vi "Generate data string.vi"(7 "New file":bool, 10 "Speed window data":T1, 11 "Timestamp at trial start":timestamp) -> (1 "Data String":string, 3 "Timestamp at trial start":timestamp)   [LabVIEW 2020]
uses:
  Typedefs/Speed window notifier data.ctl
  Typedefs/Speed logging states enum.ctl
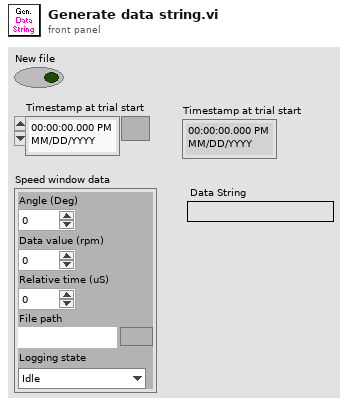
[diagram p1: front panel]
types:
  T1 = typedef "Speed window notifier data.ctl" = cluster{"Angle (Deg)":dbl, "Data value (rpm)":dbl, "Relative time (uS)":i32, "File path":path, "Logging state":T2}
  T2 = typedef "Speed logging states enum.ctl" = enum16{"Idle", "Open file", "Log", "Close file"}
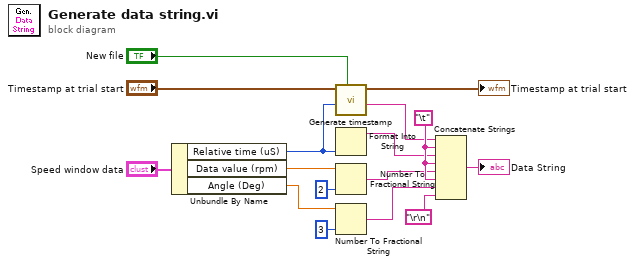
[diagram p0: block diagram]
diagram:
  w15 = "\t" ("string")
  n1 = Unbundle By Name("Speed window data") -> ("Relative time (uS)"=w5:i32, "Data value (rpm)"=w10:dbl, "Angle (Deg)"=w14:dbl)
  n2 = call "Generate timestamp.vi"("New file"="New file", "Time since acquisition start (us)"=w5, "Timestamp at trial start"="Timestamp at trial start") -> ("Date-time string (micro-second precision)"=w4:string, "Timestamp at trial start"=→"Timestamp at trial start":timestamp)  [unwired: 7 in]
  n3 = Format Into String(w5) -> (resulting string=w11:string)  [unwired: 3 in, 1 out]
  n4 = Number To Fractional String(number=w10, precision (6)=i16 2) -> (F-format string=w12:string)  [unwired: 2 in]
  n5 = Number To Fractional String(number=w14, precision (6)=i16 3) -> (F-format string=w16:string)  [unwired: 2 in]
  n6 = Concatenate Strings(w4, w15, w11, w15, w12, w15, w16, "\r\n" ("string")) -> (→"Data String":string)
